vi "FPGA_Spiral.vi"() -> ()   [LabVIEW 2010]
uses:
  <vilib>/Platform/TimedLoop/XDataNode/XDataNode.xnode
  <vilib>/Platform/TimedLoop/XDataNode/nitl_modes.ctl
  <vilib>/Platform/TimedLoop/XDataNode/XDNodeRunTimeDep.lvlib
  <vilib>/Platform/TimedLoop/XDataNode/wakeup.ctl
  <vilib>/Platform/TimedLoop/XDataNode/timing_clust.ctl
  FPGA_Typedefs/DAC_voltage_cluster.ctl
  FPGA_Typedefs/DAC_values_cluster.ctl
  FPGA_Typedefs/FPGA Cycle Counters XY.ctl
  FPGA_Typedefs/channels_array.ctl
  FPGA_Typedefs/FPGA Cycle Counters.ctl
  FPGA_Typedefs/FPGA Scan Counters.ctl
  FPGA_Typedefs/FPGA Cycle Parameters XY.ctl
  FPGA_Typedefs/FPGA Cycle Parameters.ctl
  FPGA_Typedefs/FPGA Scan Parameters.ctl
  FPGA_Typedefs/pixel_to_host_enum.ctl
panel:
  out "max pixel no.":i64
  in  "pixel-to-host mode":T1=enum."two-channel mode"
  out "Scanning?":bool
  in  "FPGA Scan Parameters":T2={"No. of waveforms"=10, "Continuous scanning"=TRUE}
  in  "Enable ADC clock?":bool=TRUE
  in  "converter box version":i16=2 min=1 max=2
  in  "ADC clock phase":u8
  out "integrated pixel values":T3
  out "data read":T3
  out "FIFO overflow":bool
  out "current pixel no.":i64
  in  "channel offsets":T3
  in  "cycles per pixel":u32=100
  in  "Scan":bool
  in  "wait for trigger?":bool
  in  "stop acquisition at FIFO overflow?":bool
  out "Acquiring?":bool
  in  "FPGA Cycle Parameters XY":T4={"FPGA Cycle Parameters X"={"Imaging cycles"=285714, "Settling cycles"=71429, "Resting cycles"=42857, "Phase advance per cycle"=0.0001399517059326172, "Imaging Multiplier advance per cycle"=0.00286865234375, "Settling Multiplier advance per cycle"=-0.0057373046875, "Imaging Initial Multiplier"=0.0, "Initial Phase"=0.0}, "FPGA Cycle Parameters Y"={"Imaging cycles"=285714, "Settling cycles"=71429, "Resting cycles"=42857, "Phase advance per cycle"=0.0001399517059326172, "Imaging Multiplier advance per cycle"=0.00286865234375, "Settling Multiplier advance per cycle"=-0.0057373046875, "Imaging Initial Multiplier"=0.0, "Initial Phase"=0.0}}
  out "DAC values to write out":T6 {"bit index" min=-1 max=17 step=1; "channel index" max=7 step=1; "offset" max=4095; "DAC voltage"."ch1" max=4095 step=1; "DAC voltage"."ch0" max=4095 step=1}
  out "In Range?":bool
  in  "Reset DAC":bool
  in  "Stop FPGA":bool
  # "Waveform generation"
  # "Pixel acquisition"
  # "Clock options"
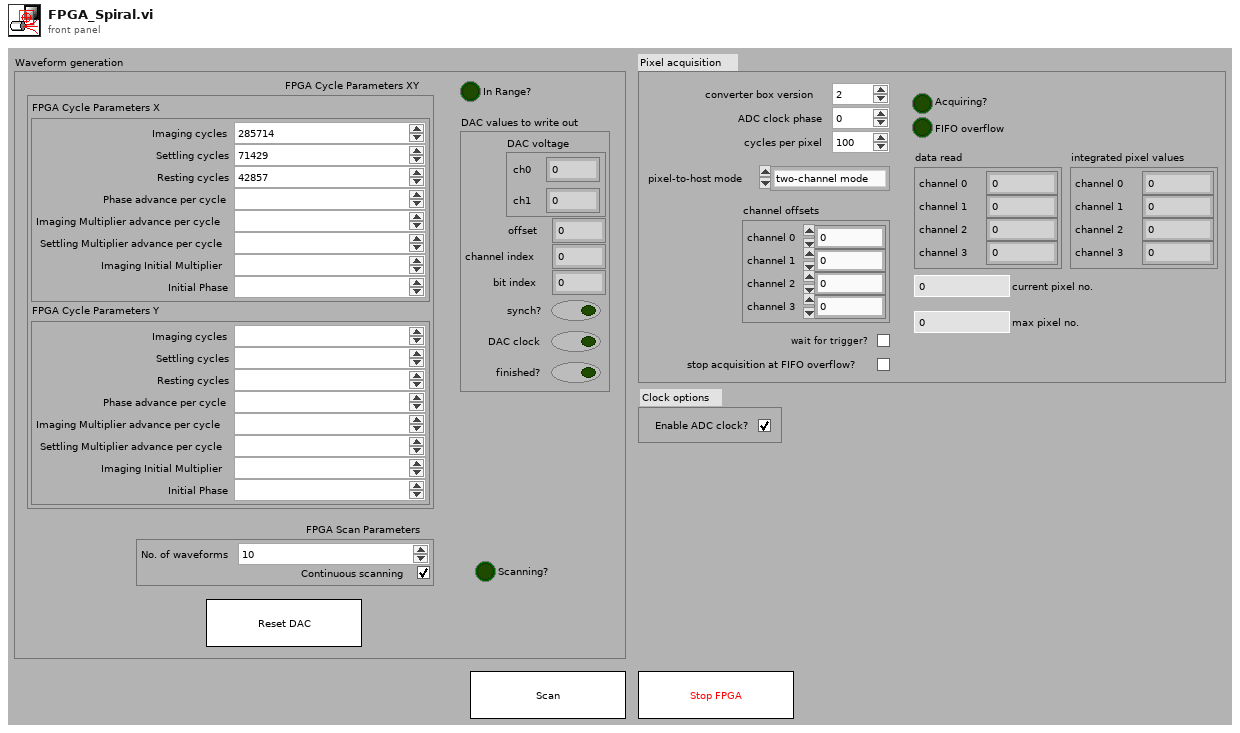
[diagram p1: front panel]
types:
  T1 = typedef "pixel_to_host_enum.ctl" = enum16{"four-channel mode", "two-channel mode"}
  T2 = typedef "FPGA Scan Parameters.ctl" = cluster{"No. of waveforms":u16, "Continuous scanning":bool}
  T3 = typedef "channels_array.ctl" = cluster{"channel 0":u32, "channel 1":u32, "channel 2":u32, "channel 3":u32}
  T4 = typedef "FPGA Cycle Parameters XY.ctl" = cluster{"FPGA Cycle Parameters X":T5, "FPGA Cycle Parameters Y":T5}
  T5 = typedef "FPGA Cycle Parameters.ctl" = cluster{"Imaging cycles":i32, "Settling cycles":i32, "Resting cycles":i32, "Phase advance per cycle":fxp<+,32,0>, "Imaging Multiplier advance per cycle":fxp<+/-,32,0>, "Settling Multiplier advance per cycle":fxp<+/-,32,0>, "Imaging Initial Multiplier":fxp<+/-,43,12>, "Initial Phase":fxp<+,32,1>}
  T6 = typedef "DAC_values_cluster.ctl" = cluster{"DAC voltage":T7, "offset":u16, "channel index":u16, "bit index":i32, "synch?":bool, "DAC clock":bool, "finished?":bool}
  T7 = typedef "DAC_voltage_cluster.ctl" = cluster{"ch0":u16, "ch1":u16}
  T8 = typedef "FPGA Cycle Counters XY.ctl" = cluster{"FPGA Cycle Counters X":T9, "FPGA Cycle Counters Y":T9}
  T9 = typedef "FPGA Cycle Counters.ctl" = cluster{"Imaging counter":i32, "Settling counter":i32, "Resting counter":i32, "Phase":fxp<+,32,1>, "Multiplier":fxp<+/-,43,12>}
  T10 = typedef "FPGA Scan Counters.ctl" = cluster{"Current part of waveform":u8, "Current waveform":u16}
  T11 = typedef "XDNodeRunTimeDep.lvlib/timing_clust.ctl" = cluster{"Expected End [f-1]":u64, "Actual End [f-1]":u64, "Finished Late? [f-1]":bool, "Expected End [i-1]":u64, "Actual End [i-1]":u64, "Finished Late? [i-1]":bool, "Expected Start [i]":u64, "Actual Start [i]":u64, "Expected Start [f]":u64, "Actual Start [f]":u64, "Source Name":string, "Structure Name":string, "Period":i64, "Deadline":i64, "Offset":i64, "Start":i64, "Priority":i32, "Timeout":i32, "Mode":T12, "Wakeup Reason":T13, "Error":errorcluster, "Source Type":string, "Secondary Source Type":string, "Global End Time":u64, "Global Start Time":u64, "Frame Duration":u64, "Iteration Duration":u64, "Assigned CPU":i32, "I/O Scan Engine Mode":u32}
  T12 = typedef "XDNodeRunTimeDep.lvlib/nitl_modes.ctl" = enum32{"No Change", "Process missed periods, maintain original phase", "Discard missed periods, maintain original phase", "Process missed periods, ignore original phase", "Discard missed periods, ignore original phase"}
  T13 = typedef "XDNodeRunTimeDep.lvlib/wakeup.ctl" = enum32{"Normal", "Aborted", "Asynchronous wakeup", "Timing source error", "Timed loop error", "Timeout"}
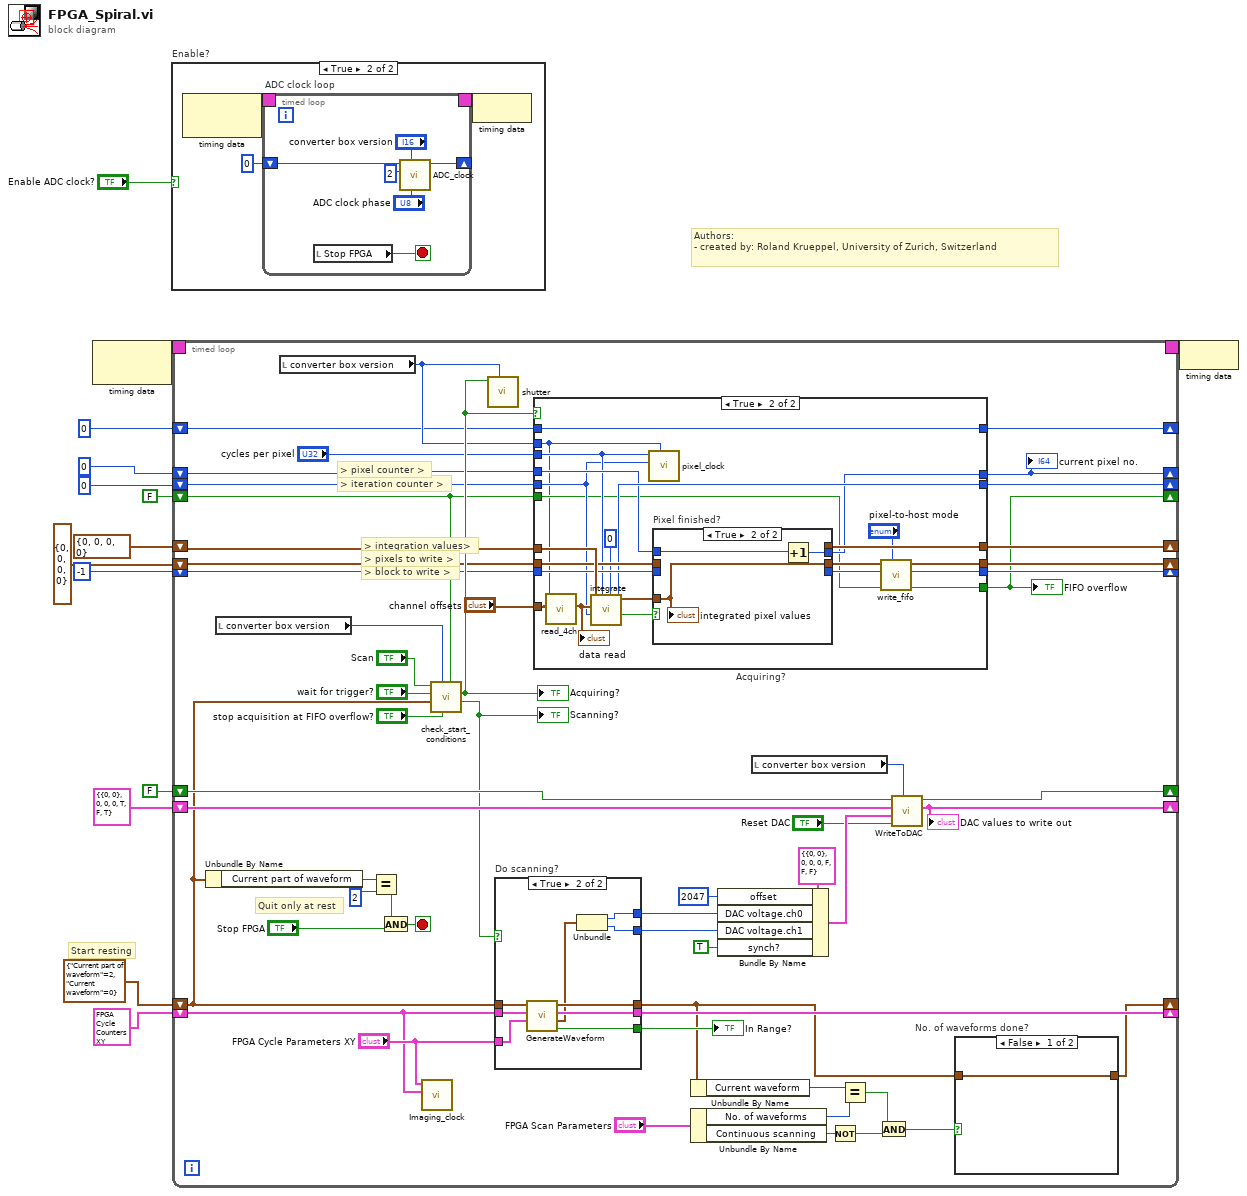
[diagram p0: block diagram]
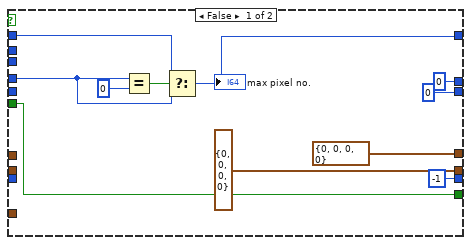
[diagram p3: hidden frame]
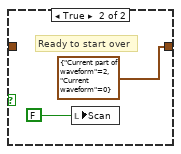
[diagram p5: hidden frame]
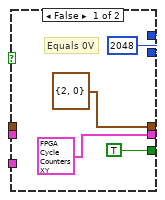
[diagram p6: hidden frame]
diagram:
  # "Authors: \n- created by: Roland Krueppel, University of Zurich, Switzerland"
  # "Start resting"
  n1 = node-c288() -> (w14:T11)  [unwired: 1 in]
  n2 = case "Enable?" shown="True" "Enable ADC clock?" {
    frame False {
    }
    frame True {
      n3 = node-c288() -> (w17:T11)  [unwired: 1 out]
      n4 = timed-loop "ADC clock loop" {
        timing: w17 -> [_]
        timing-out: [_] -> w16
        shift-right: [w22] -> _
        shift-left: u8 0 ("counter out") -> [w23]
        stop <- w18 stop-if-true
        n5 = local read "Stop FPGA"() -> (w18:bool)
        n6 = call "ADC_clock.vi"("phase"="ADC clock phase", "converter box version"="converter box version", "iterations per cycle"=u8 2, "counter in"=w23) -> ("counter out"=w22:u8)  [unwired: 7 in]
      }
      n7 = node-c288(w16) -> ()
    }
  }
  n8 = timed-loop {
    timing: w14 -> [_]
    timing-out: [_] -> w13
    shift-right: [w78] -> _
    shift-left: T6 {"DAC voltage"={"ch0"=0, "ch1"=0}, "offset"=0, "channel index"=0, "bit index"=0, "synch?"=TRUE, "DAC clock"=FALSE, "finished?"=TRUE} ("DAC values to write out") -> [w76]
    shift-right: [w77] -> _
    shift-left: FALSE ("DAC Reset out") -> [w47]
    shift-right: [w44] -> _
    shift-left: T8 {"FPGA Cycle Counters X"={"Imaging counter"=0, "Settling counter"=0, "Resting counter"=0, "Phase"=0.0, "Multiplier"=0.0}, "FPGA Cycle Counters Y"={"Imaging counter"=0, "Settling counter"=0, "Resting counter"=0, "Phase"=0.0, "Multiplier"=0.0}} ("FPGA Cycle Counters XY In") -> [w30]
    shift-right: [w62] -> _
    shift-left: T3 {"channel 0"=0, "channel 1"=0, "channel 2"=0, "channel 3"=0} ("new pixel values out") -> [w61]
    shift-right: [w59] -> _
    shift-left: -1 ("block index out") -> [w57]
    shift-right: [w60] -> _
    shift-left: T3 {"channel 0"=0, "channel 1"=0, "channel 2"=0, "channel 3"=0} ("channels out") -> [w58]
    shift-right: [w54] -> _
    shift-left: FALSE ("FIFO overflow out") -> [w51]
    shift-right: [w55] -> _
    shift-left: u32 0 ("iteration counter out") -> [w52]
    shift-right: [w56] -> _
    shift-left: i64 0 -> [w53]
    shift-right: [w40] -> _
    shift-left: T10 {"Current part of waveform"=2, "Current waveform"=0} ("FPGA Scan Counters In") -> [w35]
    shift-right: [w28] -> _
    shift-left: i64 0 -> [w29]
    stop <- w43 stop-if-true
    # "Quit only at rest"
    # "> pixel counter >"
    # "> block to write >"
    # "> integration values>"
    # "> pixels to write >"
    # "> iteration counter >"
    n9 = Unbundle By Name(w35) -> ("Current part of waveform"=w34:u8)
    n10 = local read "converter box version"() -> (w38:i16)
    n11 = local read "converter box version"() -> (w39:i16)
    n12 = Equal?(x=w34, y=u8 2) -> (x = y?=w32:bool)
    n13 = And(x=w32, y="Stop FPGA") -> (x .and. y?=w43:bool)
    n14 = call "Imaging_clock.vi"("FPGA Cycle Counters XY"=w30, "FPGA Cycle Parameters XY"="FPGA Cycle Parameters XY") -> ()  [unwired: 7 in, 1 out]
    n15 = call "check_start_conditions.vi"("FIFO overflow?"=w51, "stop at FIFO overflow?"="stop acquisition at FIFO overflow?", "converter box version"=w38, "FPGA Scan Counters"=w35, "wait for trigger?"="wait for trigger?", "Scan"="Scan") -> ("Scanning?"=w36:bool, "acquire?"=w67:bool)  [unwired: 4 in]
    "Acquiring?" <- w67
    "Scanning?" <- w36
    n16 = call "shutter.vi"("converter box version"=w39, "open?"=w67) -> ()  [unwired: 10 in]
    n17 = case "Do scanning?" shown="True" w36 {
      tunnel: w30 -> [_ w137]
      tunnel: [w129 w131] -> w75
      tunnel: [w129 w130] -> w74
      tunnel: "FPGA Cycle Parameters XY" -> [_ w136]
      tunnel: [T8 {"FPGA Cycle Counters X"={"Imaging counter"=0, "Settling counter"=0, "Resting counter"=0, "Phase"=0.0, "Multiplier"=0.0}, "FPGA Cycle Counters Y"={"Imaging counter"=0, "Settling counter"=0, "Resting counter"=0, "Phase"=0.0, "Multiplier"=0.0}} ("FPGA Cycle Counters XY In") w134] -> w44
      tunnel: [TRUE w133] -> w69
      tunnel: w35 -> [_ w138]
      tunnel: [T10 {"Current part of waveform"=2, "Current waveform"=0} ("FPGA Scan Counters In") w135] -> w41
      frame False {
        w129 = u16 2048 ("Coerced X")
        # "Equals 0V"
      }
      frame True {
        n18 = call "GenerateWaveform.vi"("FPGA Cycle Parameters XY"=w136, "FPGA Cycle Counters XY In"=w137, "FPGA Scan Counters In"=w138) -> ("In Range"=w133:bool, "Waveform Out"=w132:cluster{"Coerced Out":u16, "Coerced Out":u16}, "FPGA Cycle Counters XY Out"=w134:T8, "FPGA Scan Counters Out"=w135:T10)  [unwired: 1 in]
        n19 = Unbundle(w132) -> ("Coerced Out"=w131:u16, "Coerced Out"=w130:u16)
      }
    }
    "In Range?" <- w69
    n20 = case "Acquiring?" shown="True" w67 {
      tunnel: [T3 {"channel 0"=0, "channel 1"=0, "channel 2"=0, "channel 3"=0} ("new pixel values out") w110] -> w62
      tunnel: w61 -> [_ w115]
      tunnel: [T3 {"channel 0"=0, "channel 1"=0, "channel 2"=0, "channel 3"=0} ("channels out") w114] -> w60
      tunnel: w58 -> [_ w107]
      tunnel: [-1 ("block index out") w113] -> w59
      tunnel: w57 -> [_ w109]
      tunnel: w52 -> [_ w98]
      tunnel: [u32 0 ("iteration counter out") w105] -> w55
      tunnel: [w92 w96] -> w54
      tunnel: w53 -> [w82 w103]
      tunnel: [i64 0 w102] -> w56
      tunnel: "channel offsets" -> [_ w100]
      tunnel: "cycles per pixel" -> [_ w99]
      tunnel: w51 -> [w92 w97]
      tunnel: w39 -> [_ w95]
      tunnel: w29 -> [w83 w93]
      tunnel: [w86 w93] -> w28
      frame False {
        n21 = Equal?(x=w82, y=i64 0) -> (x = y?=w84:bool)
        n22 = Select(t=w83, s=w84, f=w82) -> (s? t:f=w86:i64)
        "max pixel no." <- w86
      }
      frame True {
        n23 = call "read_4ch.vi"("channel offsets"=w100, "converter box version"=w95) -> ("read output"=w111:T3)  [unwired: 9 in]
        "data read" <- w111
        n24 = call "integrate.vi"("waiting iterations per pixel"=u32 0, "integration iterations per pixel"=w99, "iteration counter in"=w98, "sampling values in"=w111, "previous pixel values in"=w115) -> ("finished?"=w104:bool, "iteration counter out"=w105:u32, "new pixel values out"=w112:T3)  [unwired: 4 in]
        n25 = call "pixel_clock.vi"("converter box version"=w95, "current iteration"=w98, "iterations per pixel"=w99) -> ()  [unwired: 9 in]
        n26 = case "Pixel finished?" shown="True" w104 {
          tunnel: w112 -> [w119 w122]
          tunnel: [w119 _] -> w110
          tunnel: w109 -> [w118 _]
          tunnel: [w118 _] -> w108
          tunnel: w107 -> [w117 _]
          tunnel: [w117 w122] -> w106
          tunnel: w103 -> [w116 w121]
          tunnel: [w116 w120] -> w102
          frame False {
          }
          frame True {
            n27 = Increment(x=w121) -> (x+1=w120:i64)
            "integrated pixel values" <- w122
          }
        }
        n28 = call "write_fifo.vi"("pixel-to-host\n mode"="pixel-to-host mode", "FIFO overflow in"=w97, "block index in"=w108, "values to be written"=w106) -> ("FIFO overflow out"=w96:bool, "block index out"=w113:i32, "channels out"=w114:T3)  [unwired: 5 in]
      }
    }
    "FIFO overflow" <- w54
    "current pixel no." <- w56
    n29 = Unbundle By Name(w41) -> ("Current waveform"=w49:u16)
    n30 = Unbundle By Name("FPGA Scan Parameters") -> ("No. of waveforms"=w73:u16, "Continuous scanning"=w72:bool)
    n31 = Bundle By Name(cluster=T6 {"DAC voltage"={"ch0"=0, "ch1"=0}, "offset"=0, "channel index"=0, "bit index"=0, "synch?"=FALSE, "DAC clock"=FALSE, "finished?"=FALSE} ("New DAC values generated"), "offset"=u16 2047, "DAC voltage.ch0"=w75, "DAC voltage.ch1"=w74, "synch?"=TRUE) -> (w79:T6)
    n32 = local read "converter box version"() -> (w48:i16)
    n33 = Not(x=w72) -> (.not. x?=w71:bool)
    n34 = Equal?(x=w49, y=w73) -> (x = y?=w70:bool)
    n35 = And(x=w70, y=w71) -> (x .and. y?=w68:bool)
    n36 = call "WriteToDAC.vi"("converter box version"=w48, "DAC New Reset"="Reset DAC", "New DAC values generated"=w79, "DAC values to write In"=w76, "DAC Reset State In"=w47) -> ("DAC values to write out"=w78:T6, "DAC Reset State out"=w77:bool)  [unwired: 2 in]
    "DAC values to write out" <- w78
    n37 = case "No. of waveforms done?" shown="False" w68 {
      tunnel: w41 -> [w123 _]
      tunnel: [w123 T10 {"Current part of waveform"=2, "Current waveform"=0} ("FPGA Scan Counters In")] -> w40
      frame False {
      }
      frame True {
        # "Ready to start over"
        n38 = local write "Scan"(FALSE ("Do Scanning")) -> ()
      }
    }
  }
  n39 = node-c288(w13) -> ()
